vi "Write Units.vi"(8 "error in (no error)":errorcluster, 10 "Units":string, 11 "Abs_Numeric in":refnum<class "Abs_Numeric.lvclass">) -> (0 "error out":errorcluster, 3 "Abs_Numeric out":refnum<class "Abs_Numeric.lvclass">)   [LabVIEW 2021, in "Abs_Numeric.lvclass"]
uses:
  Abs_Numeric.lvclass
  Abs_Numeric.lvclass/Abs_Numeric.ctl
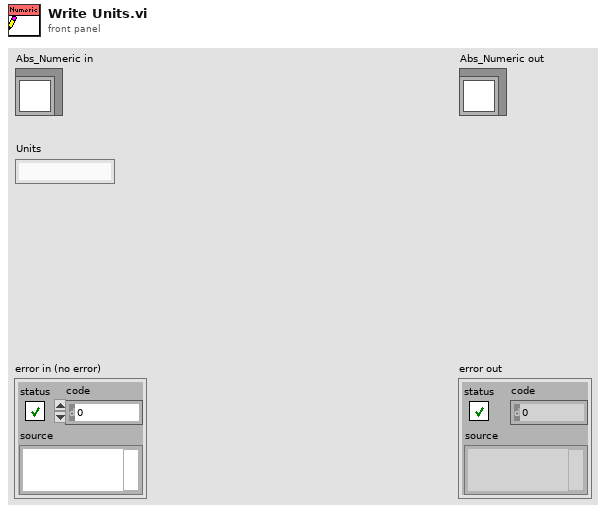
[diagram p1: front panel]
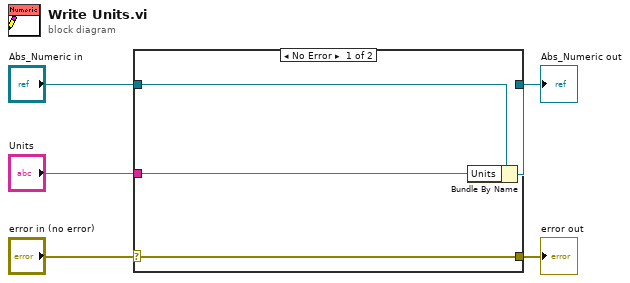
[diagram p0: block diagram]
diagram:
  n1 = case shown="No Error" "error in (no error)" {
    selector: "error in (no error)" -> [w9 w10]
    tunnel: [w9 w10] -> w4
    tunnel: [w7 w11] -> w2
    tunnel: "Abs_Numeric in" -> [w8 w11]
    tunnel: "Units" -> [w6 _]
    frame No Error {
      n2 = Bundle By Name(cluster=w8, "Units"=w6) -> (w7:refnum<class "Abs_Numeric.lvclass">)
    }
    frame Error {
    }
  }
  "error out" <- w4
  "Abs_Numeric out" <- w2
